vi "OCR_FOV.vi"(3 "error in":errorcluster, 4 "Size factor":dbl, 5 "Image in":T1) -> (0 "error out":errorcluster, 1 "FOV":dbl, 2 "Image out":T1(plugin-control))   [LabVIEW 2015]
uses:
  <vilib>/vision/Image Controls.llb/IMAQ Image.ctl
  <vilib>/vision/NI_Vision_Development_Module.lvlib
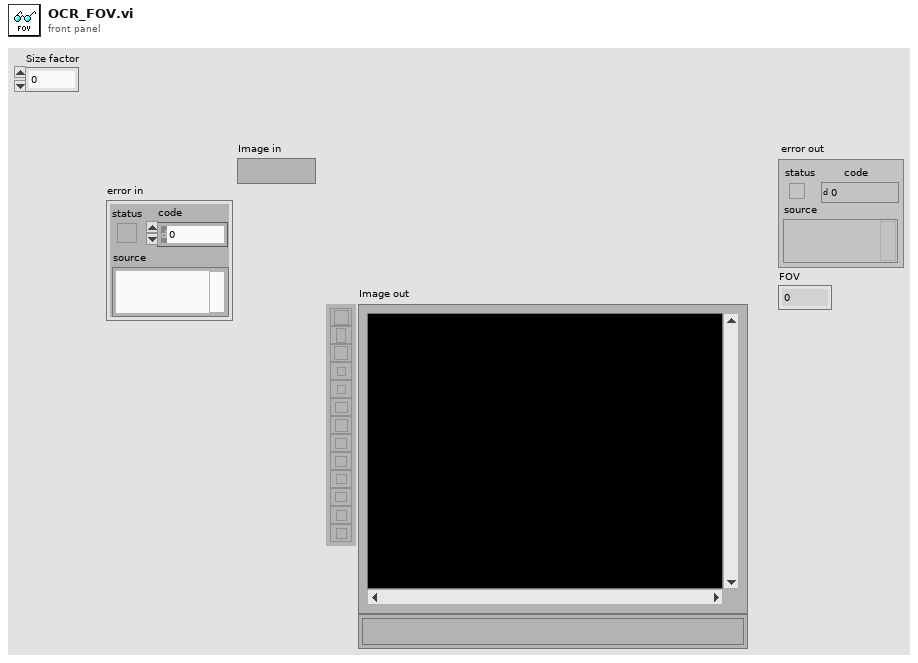
[diagram p1: front panel]
types:
  T1 = typedef "IMAQ Image.ctl" = refnum<image>
  T2 = cluster{"Dark Characters":bool, "Number of Blocks":i32, "Threshold Limits":cluster{"Lower Value":i32, "Upper Value":i32}, "Optimize For Speed":bool, "Perform Bi-modal Calculation":bool}
  T3 = typedef "IMAQ Rectangle" = cluster{"Left":i32, "Top":i32, "Right":i32, "Bottom":i32, "Rotation":dbl}
  T4 = typedef "IMAQ OCR Session.ctl" = refnum<k1>
  T5 = cluster{"Left":i32, dbl, dbl, dbl, "Rotation":dbl}
  T6 = typedef "ROI Descriptor" = cluster{"Global Rectangle":i32[], "Contours":cluster{"ID":enum32{"External", "Internal"}, "Type":u32, "Coordinates":i32[]}[]}
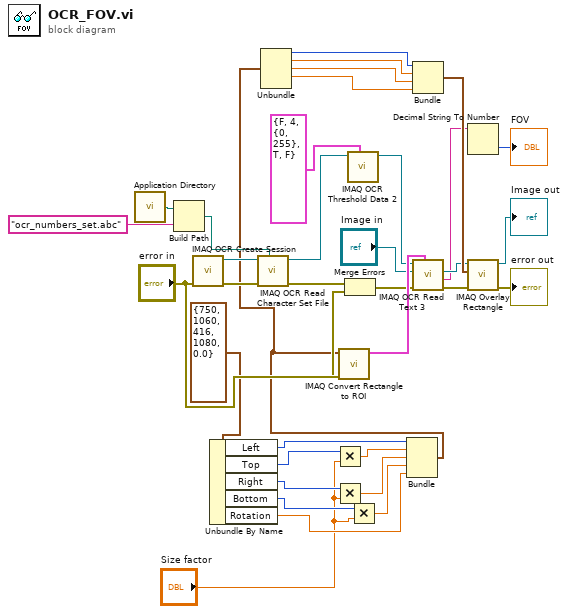
[diagram p0: block diagram]
diagram:
  n1 = call <vilib>:"Application Directory.vi"() -> ("Application Directory"=w24:path)
  n2 = Build Path(base path=w24, name or relative path="ocr_numbers_set.abc") -> (appended path=w22:path)
  n3 = call "IMAQ OCR Create Session"("error in (no error)"="error in") -> ("error out"=w20:errorcluster, "IMAQ OCR Session"=w35:T4)  [unwired: 9 out]
  n4 = Unbundle By Name(T3 {"Left"=750, "Top"=1060, "Right"=416, "Bottom"=1080, "Rotation"=0.0} ("Rectangle")) -> ("Left"=w6:i32, "Top"=w5:i32, "Right"=w11:i32, "Bottom"=w4:i32, "Rotation"=w10:dbl)
  n5 = call "IMAQ OCR Read Character Set File"("File Path"=w22, "error in (no error)"=w20, "IMAQ OCR Session"=w35) -> ("error out"=w19:errorcluster, "IMAQ OCR Session (dup)"=w28:T4)  [unwired: 2 in, 5 out]
  n6 = Multiply(x=w5, y="Size factor") -> (x*y=w2:dbl)
  n7 = Multiply(x=w11, y="Size factor") -> (x*y=w7:dbl)
  n8 = call-poly "IMAQ OCR Threshold Data 2"("Threshold Data"=T2 {"Dark Characters"=FALSE, "Number of Blocks"=4, "Threshold Limits"={"Lower Value"=0, "Upper Value"=255}, "Optimize For Speed"=TRUE, "Perform Bi-modal Calculation"=FALSE}, "IMAQ OCR Session"=w28) -> ("IMAQ OCR Session (dup)"=w27:T4)  [unwired: 5 in, 4 out]
  n9 = Multiply(x=w4, y="Size factor") -> (x*y=w1:dbl)
  n10 = Bundle("Left"=w6, w2, w7, w1, "Rotation"=w10) -> (w8:T5)  [unwired: 1 in]
  n11 = Unbundle(w8) -> ("Left"=w34:i32, w33:dbl, w32:dbl, w31:dbl)  [unwired: 1 out]
  n12 = call "IMAQ Convert Rectangle to ROI"("error in (no error)"="error in", "Rectangle"=w8) -> ("error out"=w12:errorcluster, "ROI Descriptor"=w36:T6)  [unwired: 7 in]
  n13 = Merge Errors(w19, w12) -> (w18:errorcluster)
  n14 = Bundle("Left"=w34, w33, w32, w31) -> (w30:cluster{"Left":i32, dbl, dbl, dbl})  [unwired: 1 in]
  n15 = call "IMAQ OCR Read Text 3"("ROI Descriptor"=w36, "error in (no error)"=w18, "Image"="Image in", "IMAQ OCR Session"=w27) -> ("error out"=w17:errorcluster, "Read String"=w15:string, "Image (dup)"=w25:T1)  [unwired: 1 in, 4 out]
  n16 = Decimal String To Number(string=w15) -> (number=→"FOV":i32)  [unwired: 2 in, 1 out]
  n17 = call "IMAQ Overlay Rectangle"("error in (no error)"=w17, "Rectangle"=w30, "Image"=w25) -> ("error out"=→"error out":errorcluster, "Image Out"=→"Image out":T1)  [unwired: 7 in]
